vi "Init Msg.vi"(10 "Msg Input":refnum<class "Msg Input.lvclass">) -> (2 "Msg":refnum<class "Msg.lvclass">)   [LabVIEW 2020, in "jettl.lvlib" / "Stop jettl Msg.lvlib" / "Stop Msg.lvlib"]
uses:
  Stop Msg.lvlib
  Msg Input/Msg Input.lvclass
  Msg/Msg.lvclass
  Stop Msg/Stop Msg.lvclass
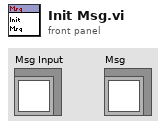
[diagram p1: front panel]
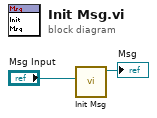
[diagram p0: block diagram]
diagram:
  n1 = call "Init Msg.vi"("Msg Input"="Msg Input") -> ("Stop Msg out"=→"Msg":refnum<class "Stop Msg.lvclass">)  [unwired: 10 in]
